vi "HB_PollingAgent.appendData2Variant.vi"(0 "initData":variant, 2 "Question":string="Undefinierte Umfrage!", 5 "error in (no error)":errorcluster) -> (14 "dup initData":variant, 19 "error out":errorcluster)   [LabVIEW 2009, in "HB_PollingAgent.lvlib" / "HB_PollingAgent.lvclass"]
uses:
  HB_PollingAgent.lvclass
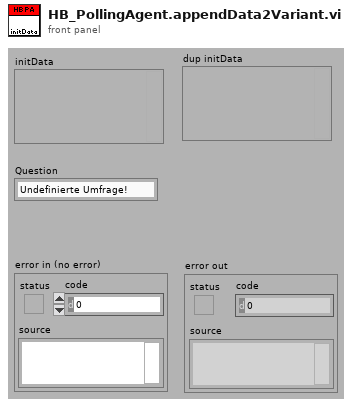
[diagram p1: front panel]
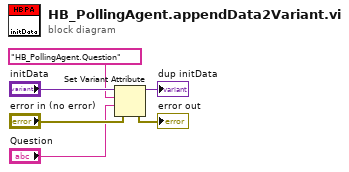
[diagram p0: block diagram]
diagram:
  n1 = Set Variant Attribute(Variant="initData", name="HB_PollingAgent.Question", value="Question", error in="error in (no error)") -> (Variant out=→"dup initData":variant, error out=→"error out":errorcluster)  [unwired: 1 out]
